vi "Init.vi"(0 "reference in":refnum<class "FPGA_Mock.lvclass">, 11 "error in (no error)":errorcluster) -> (4 "reference out":refnum<class "FPGA_Mock.lvclass">, 15 "error out":errorcluster)   [LabVIEW 2019, in "FPGA_Mock.lvclass"]
uses:
  FPGA_Mock.lvclass
  SharedData.ctl
  FPGA_Mock.lvclass/FPGA_Mock.ctl
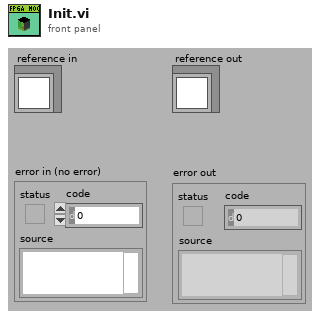
[diagram p1: front panel]
types:
  T1 = typedef "FPGA_Mock.lvclass/SharedData.ctl" = cluster{"DI":bool[], "DO":bool[], "AO":dbl[]}
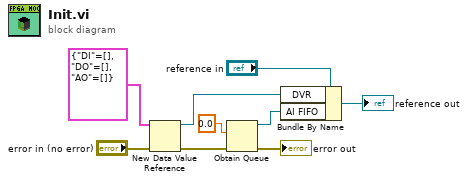
[diagram p0: block diagram]
diagram:
  n1 = New Data Value Reference(data value=T1 {"DI"=[], "DO"=[], "AO"=[]} ("SharedData"), error in="error in (no error)") -> (data value reference=w6:refnum<data-value>, error out=w3:errorcluster)
  n2 = Obtain Queue(element data type=0.0, error in (no error)=w3) -> (queue out=w4:refnum<queue>, error out=→"error out":errorcluster)  [unwired: 3 in, 1 out]
  n3 = Bundle By Name(cluster="reference in", "DVR"=w6, "AI FIFO"=w4) -> (→"reference out":refnum<class "FPGA_Mock.lvclass">)
